vi "Verify as JSON.vi"(5 "Label":string, 7 "Options":refnum<class "Options.lvclass">, 8 "error in":errorcluster, 10 "Anything":variant, 11 "TestCase in":refnum<class "TestCase.lvclass">) -> (0 "error out":errorcluster, 3 "TestCase out":refnum<class "TestCase.lvclass">)   [LabVIEW 2026, in "VITester.Extension.lvlib"]
doc: "Takes in anything. Flattens it to JSON."
uses:
  VITester.Extension.lvlib
  <vilib>/Addons/_JKI Toolkits/VI Tester/TestCase.llb/TestCase.lvclass
  Approval Tests/Options/Options.lvclass
  Approval Tests/Options/Options.lvclass/Options.ctl
  Approval Tests/Naming Data/Naming Data.lvclass/Naming Data.ctl
  Approval Tests/Naming Data/Read Test VI Name.vi
  Approval Tests/Naming Data/Write Test VI Name.vi
  Approval Tests/Approval Tests.lvlib
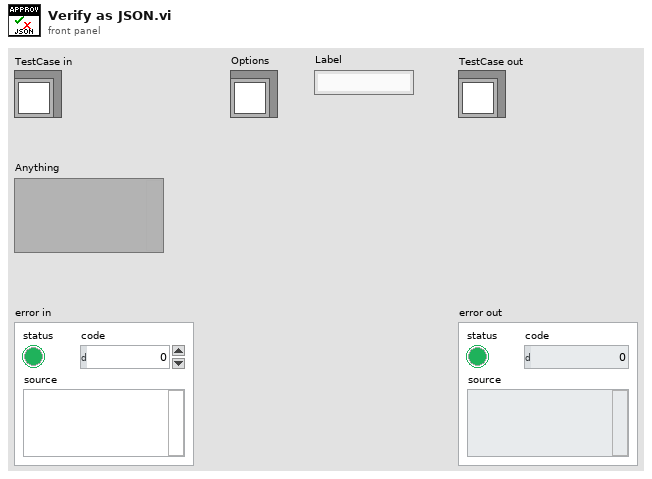
[diagram p1: front panel]
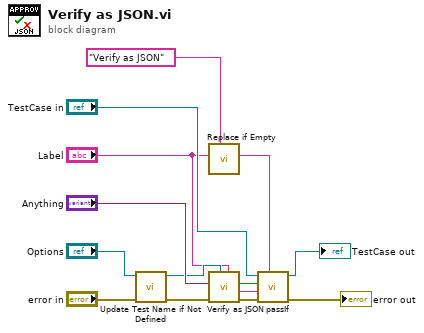
[diagram p0: block diagram]
diagram:
  n1 = call "Update Test Name if Not Defined.vi"("error in"="error in", "Options in"="Options") -> ("error out"=w11:errorcluster, "Options out"=w4:refnum<class "Options.lvclass">)  [unwired: 8 in]
  n2 = call "Replace if Empty.vi"("if empty"="Verify as JSON", "Text in"="Label") -> ("Text out"=w1:string)  [unwired: 9 in]
  n3 = call "Verify as JSON.vi"("Label"="Label", "Approval Tests.lvlib:Options.lvclass"=w4, "error in"=w11, "Anything"="Anything") -> ("error out"=w13:errorcluster, "Failure Message"=w7:string, "Passed?"=w8:bool)  [unwired: 5 in]
  n4 = call-dynamic "passIf.vi"("custom report message (\"\")"=w1, "error in (no error)"=w13, "message (\"\")"=w7, "pass"=w8, "TestCase in"="TestCase in") -> ("error out"=→"error out":errorcluster, "TestCase out"=→"TestCase out":refnum<class "TestCase.lvclass">)  [unwired: 5 in]
